vi "Obtain Host Sample Data Notifier.vi"(8 "error in (no error)":errorcluster, 10 "Create New?":bool) -> (0 "error out":errorcluster, 3 "Sample Data Notifier":refnum<notifier>)   [LabVIEW 2015, in "Tool Module.lvlib"]
uses:
  Tool Module.lvlib
  _Sample Data Rtn Cluster--typedef.ctl
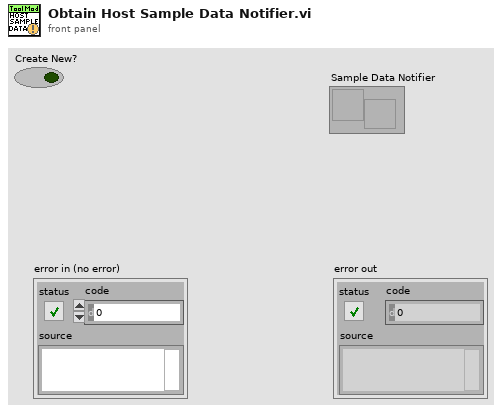
[diagram p1: front panel]
types:
  T1 = typedef "Tool Module.lvlib/_Sample Data Rtn Cluster--typedef.ctl" = cluster{"InspectCycle":bool, "Acquiring Data":bool, "Sample Available":bool, "Scan Complete":bool, "Cancelled":bool, "Scan Data Array":u32[], "error cluster":errorcluster}
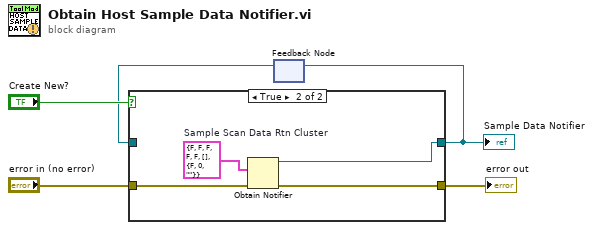
[diagram p0: block diagram]
diagram:
  n1 = feedback #1() -> (w1:refnum<notifier>)  [unwired: 1 in]
  n2 = case shown="True" "Create New?" {
    tunnel: [w7 w9] -> w2
    tunnel: "error in (no error)" -> [w6 w11]
    tunnel: [w6 w10] -> w3
    tunnel: w1 -> [w7 _]
    frame False {
    }
    frame True {
      w8 = T1 {"InspectCycle"=FALSE, "Acquiring Data"=FALSE, "Sample Available"=FALSE, "Scan Complete"=FALSE, "Cancelled"=FALSE, "Scan Data Array"=[], "error cluster"={"status"=FALSE, "code"=0, "source"=""}}  # Sample Scan Data Rtn Cluster
      n3 = Obtain Notifier(notification data type=w8, error in (no error)=w11) -> (notifier out=w9:refnum<notifier>, error out=w10:errorcluster)  [unwired: 2 in, 1 out]
    }
  }
  "error out" <- w3
  "Sample Data Notifier" <- w2
  n4 = feedback-in #1(w2) -> ()
